vi "Send Message.vi"(8 "error in":errorcluster, 9 "IMessage.lvclass":refnum<class "IMessage.lvclass">, 10 "Receiver ID":string, 11 "Copy of PCAN in":refnum<class "PCAN.lvclass">) -> (0 "error out":errorcluster, 3 "Copy of PCAN out":refnum<class "PCAN.lvclass">)   [LabVIEW 2024, in "PCAN.lvlib" / "PCAN.lvclass"]
uses:
  PCAN.lvclass
  PCAN.lvclass/PCAN.ctl
  Source/Interfaces/IMessage/IMessage.lvclass
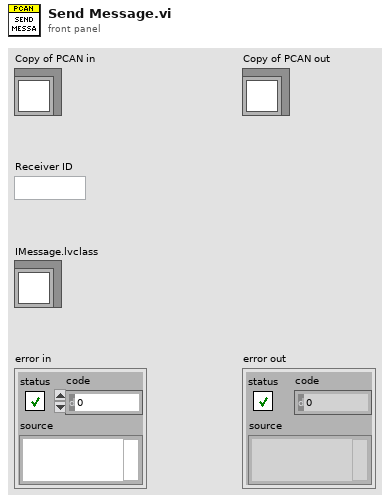
[diagram p1: front panel]
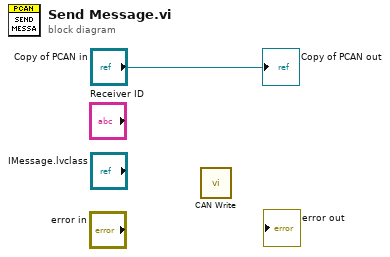
[diagram p0: block diagram]
diagram:
  n1 = call <instrlib>:"CAN Write.vi"() -> ()  [unwired: 10 in, 2 out]
  "Copy of PCAN out" <- "Copy of PCAN in"
